vi "BFP-CLAMP-baselinecorrect.vi"() -> ()   [LabVIEW 2017]
uses:
  <vilib>/userdefined/High Color/IMAQdx.ctl
  <vilib>/vision/driver/IMAQdx.llb/IMAQdx Buffer Number Mode.ctl
  <vilib>/DAQmx/write.llb/DAQmx Write (Analog DBL 1Chan 1Samp).vi
  <vilib>/Utility/file.llb/Write To Spreadsheet File (DBL).vi
  <vilib>/Utility/file.llb/Write To Spreadsheet File (string).vi
  <vilib>/DAQmx/create/channels.llb/DAQmx Create Channel (AO-Voltage-Basic).vi
  <vilib>/DAQmx/miscellaneous.llb/DAQmx Fill In Error Info.vi
  <vilib>/Utility/file.llb/Read From Spreadsheet File (DBL).vi
  <vilib>/vision/NI_Vision_Development_Module.lvlib
  <vilib>/vision/driver/NI_Vision_Acquisition_Software.lvlib
  <resource>/objmgr/imaqdx.rc
panel:
  in  "Clamp at (pN)":dbl
  in  "SD x":dbl=1.0
  out "clamp test":bool=TRUE
  out "Data":cluster{"Y":dbl[], "Y":dbl[]}[](graph)
  out "chemin complet force mean":path
  in  "box mean (pts)":i32=10
  out "chemin complet position":path
  out "test fin":bool
  out "t0":u32
  out "slow":string="prosilica-slow.icd"
  out "fast":string="prosilica.icd"
  out "derniere image":u32
  out "chemin complet force":path
  out "chemin":path caption="chemin sélectionné"
  out "# FC":i32
  out "voltage stop (V)":dbl
  out "cluster fit":T1
  out "N pas wait":i32
  out "N pas stop":i32
  in  "F contact (pN)":dbl=500.0
  in  "Measure forces":bool
  in  "Z lenght (um)":dbl=1.0
  in  "v press (um/s)":dbl=1.0
  out "t total / FC (s)":dbl
  out "# pts press":i32=500
  out "DV P753.2DV (V/um)":dbl
  in  "number A/R":i32=5
  out "step press (V)":dbl
  out "step press  (ms)":dbl
  out "V max (V)":dbl
  in  "t contact (s)":dbl
  out "t total / run (s)":dbl
  in  "t wait (s)":dbl=1.0
  in  "v pull (um/s)":dbl=1.0
  out "# pts pull":i32=500
  out "step pull  (ms)":dbl
  out "step pull (V)":dbl
  out "rectangle selection":i32[](array[numeric])
  out "calib um/pix":dbl=0.094 format="%.4f"
  in  "calibration":dbl=0.094
  out "X coord profile":dbl[](array[numeric])
  out "baseline (pN)":dbl caption="B-Line (pN)" format="%0.2f"
  out "SD noise (pN)":dbl caption="SD (pN)" format="%0.2f"
  in  "longueur fit (pts)":i32=11
  out "40x 1.5x 6.7x":dbl=3.0
  out "40x 1x 6.7x":dbl=3.0
  in  "IMAQdx MAZ":T2="cam0"
  out "Frame Rate":dbl
  out "?":T3(plugin-control)
  out "2Rc (µm)":dbl
  out "2Rg (µm)":dbl=8.0
  out "2Rp (µm)":dbl=3.0
  out "DP (cmH2O)":dbl
  in  "2Rc (pix)":dbl=1.0
  in  "2Rg (pix)":dbl=8.0
  in  "2Rp (pix)":dbl=3.0
  in  "k voulue (pN/nm)":dbl=1.0
  in  "Stop calibration":bool
  in  "sortie carte AO":tag="Dev1/ao0" caption="AO"
  in  "IMAQdx Session":T2="cam0"
  out "profil / pix":cluster{dbl[], "X Axis Averages":sgl[]}(graph)
  out "Frame Rate":dbl
  in  "Stop (F) 2":bool caption="Stop focus"
  out "FOCUSING":T3(plugin-control)
  out "ligneY (pix) <=7":i32
  out "ligne X (pix) >=200":i32
  # "Indicateurs variables locales"
  # "CALIBRATION"
  # "CAMERA"
  # "CLAMP"
  # "exposure 1 msec, gain = 24 (set in MAX)"
  # "Noise \nand Baseline\ncorrections"
  # "PIEZO"
  # ">>>"
  # "FORCE PARAMETERS"
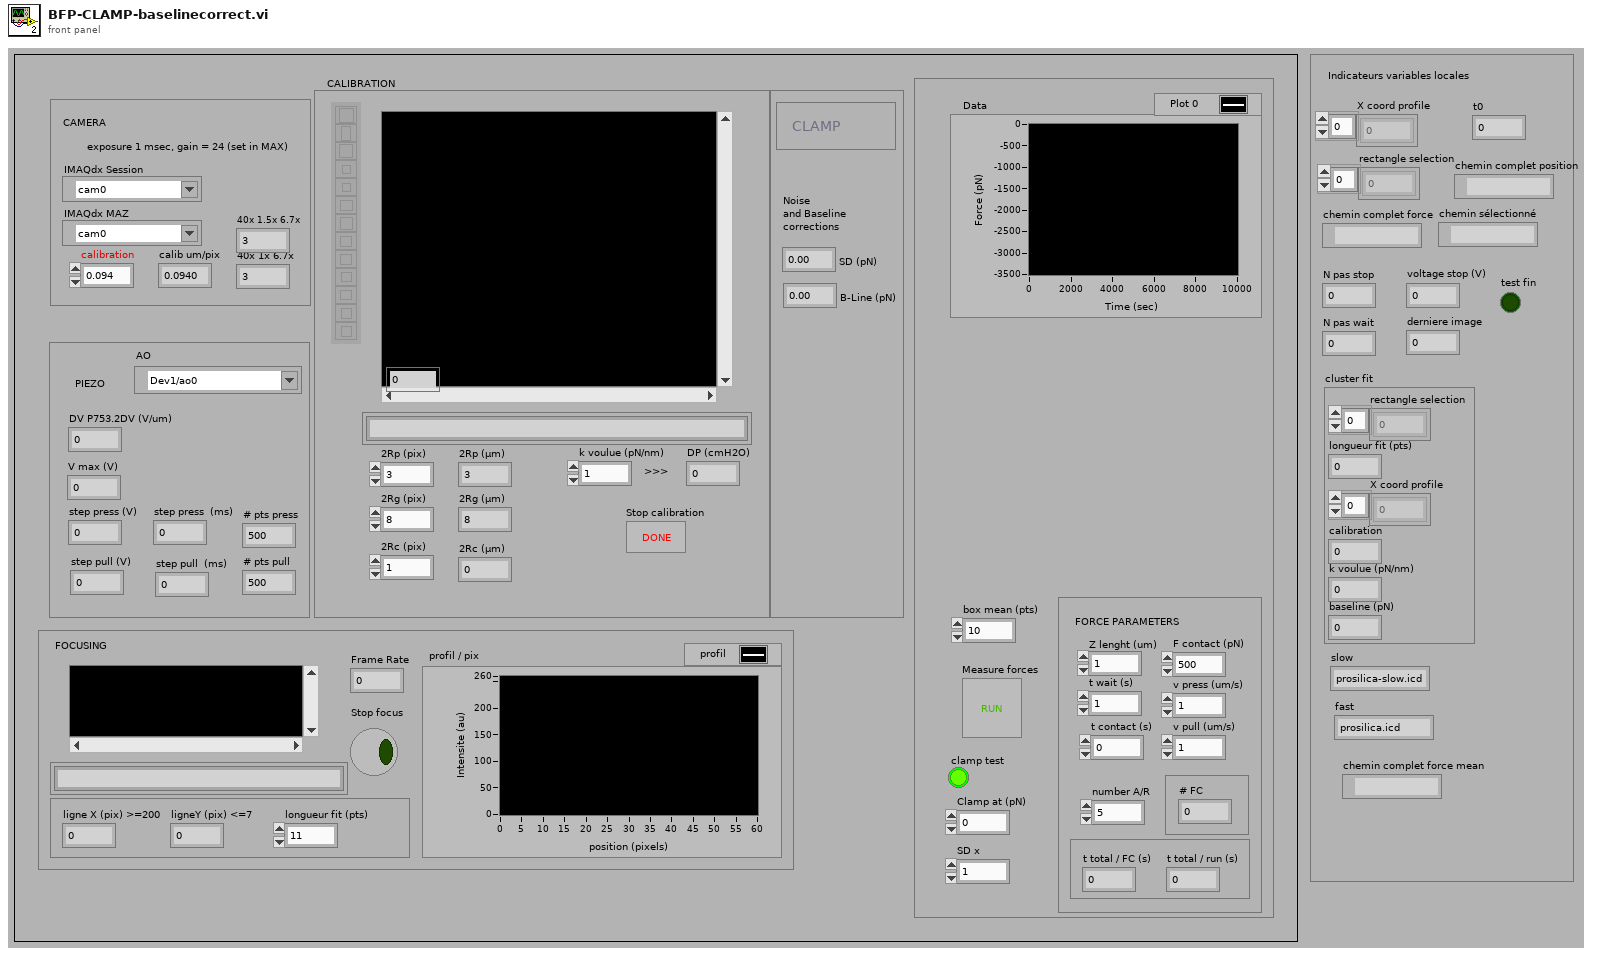
[diagram p1: front panel]
types:
  T1 = cluster{"rectangle selection":i32[], "longueur fit (pts)":i32, "X coord profile":dbl[], "calibration":dbl, "k voulue (pN/nm)":dbl, "baseline (pN)":dbl}
  T2 = typedef "IMAQdx.ctl" = refnum<k21>
  T3 = typedef "IMAQ Image.ctl" = refnum<image>
  T4 = typedef "NI_Vision_Acquisition_Software.lvlib/IMAQdx Buffer Number Mode.ctl" = enum32{"Next", "Last", "Buffer Number", "Every", "Last New"}
  T5 = typedef "IMAQ Rectangle" = cluster{"Left":i32, "Top":i32, "Right":i32, "Bottom":i32, "Rotation":dbl}
  T6 = typedef "ROI Descriptor" = cluster{"Global Rectangle":i32[], "Contours":cluster{"ID":enum32{"External", "Internal"}, "Type":u32, "Coordinates":i32[]}[]}
  T7 = cluster{"Left":i32, "Top":i32, "Right":i32, "Bottom":i32}
  T8 = cluster{"Global Rectangle[0]":i32, "Global Rectangle[1]":i32, "Global Rectangle[2]":i32, "Global Rectangle[3]":i32, "Global Rectangle[4]":i32, "Global Rectangle[5]":i32, "Global Rectangle[6]":i32, "Global Rectangle[7]":i32, "Global Rectangle[8]":i32}
  T9 = cluster{"task out":refnum<k21>, "error out":errorcluster}
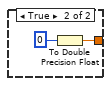
[diagram p4: hidden frame]
diagram:
  n1 = flat-sequence {
    tunnel: [w72] -> w13
    tunnel: w13 -> [w84]
    tunnel: [w161] -> w6
    tunnel: [w160] -> w4
    tunnel: [w159] -> w2
    tunnel: w6 -> [w245]
    tunnel: [w245] -> w5
    tunnel: w4 -> [w244]
    tunnel: [w244] -> w3
    tunnel: w2 -> [w243]
    tunnel: [w243] -> w1
    tunnel: w5 -> [w258]
    tunnel: w3 -> [w248]
    tunnel: w1 -> [w249]
    tunnel: [w246] -> w12
    tunnel: [w247] -> w10
    tunnel: [w250] -> w8
    tunnel: w12 -> [w270]
    tunnel: [w270] -> w11
    tunnel: w10 -> [w269]
    tunnel: [w269] -> w9
    tunnel: w8 -> [w268]
    tunnel: [w268] -> w7
    tunnel: w11 -> [w277]
    tunnel: w9 -> [w274]
    tunnel: w7 -> [w275]
    frame #0 {
      n2 = call <vilib>:"IMAQdx Open Camera.vi"("Session In"="IMAQdx MAZ") -> ("error out"=w21:errorcluster, "Session Out"=w20:T2)  [unwired: 2 in, 7 out]
      n3 = call <vilib>:"IMAQdx Read Attributes.vi"("error in"=w21, "Filename"="defaut.icd", "Session In"=w20) -> ("error out"=w19:errorcluster, "Session Out"=w24:T2)  [unwired: 7 out]
      n4 = call <vilib>:"IMAQdx Configure Grab.vi"("error in"=w19, "Session In"=w24) -> ("error out"=w16:errorcluster, "Session Out"=w17:T2)  [unwired: 1 in, 7 out]
      n5 = call <vilib>:"IMAQdx Close Camera.vi"("error in"=w16, "Session In"=w17) -> ("error out"=w18:errorcluster)  [unwired: 9 out]
      n6 = call <vilib>:"Simple Error Handler.vi"("error in (no error)"=w18) -> ()  [unwired: 1 in, 8 out]
      "40x 1x 6.7x" <- ext 0.094 ("40x 1x 6.7x")
      "40x 1.5x 6.7x" <- ext 0.0625 ("40x 1x 6.7x")
    }
    frame #1 {
      n7 = while "calibration \"evans\"" {
        stop <- w29 stop-if-true
        n8 = local write "calibration"("calibration") -> ()
        n9 = Bundle(240, 251, 440, 230) -> (w33:cluster{i32, i32, i32, i32})  [unwired: 1 out]
        n10 = Multiply(x="calibration", y="2Rc (pix)") -> (x*y=w40:dbl)
        "2Rc (µm)" <- w40
        n11 = Multiply(x="2Rp (pix)", y="calibration") -> (x*y=w44:dbl)
        "2Rp (µm)" <- w44
        n12 = Multiply(x="2Rg (pix)", y="calibration") -> (x*y=w41:dbl)
        "2Rg (µm)" <- w41
        n13 = Divide(x=1, y=1000000) -> (x/y=w66:dbl)
        n14 = Divide(x=3.141592653589793, y=2) -> (x/y=w52:dbl)
        n15 = Divide(x=1, y=1000) -> (x/y=w67:dbl)
        n16 = local write "k voulue (pN/nm)"("k voulue (pN/nm)") -> ()
        n17 = call "Vision Acquisition"("Stop (F)"="Stop calibration") -> ("Image Out"=w31:T3, "Frame Rate"=→"Frame Rate":dbl, "Stopped"=w29:bool)  [unwired: 3 in, 21 out]
        n18 = Multiply(x="k voulue (pN/nm)", y=w67) -> (x*y=w64:dbl)
        n19 = Multiply(x=w52, y=w66) -> (x*y=w65:dbl)
        n20 = Divide(x=w41, y=w40) -> (x/y=w39:dbl)
        n21 = Divide(x=w41, y=w44) -> (x/y=w43:dbl)
        n22 = Multiply(x=w44, y=w65) -> (x*y=w47:dbl)
        n23 = call "IMAQ Overlay Rectangle"("Rectangle"=w33, "Image"=w31) -> ("Image Out"=→"?":T3)  [unwired: 4 in, 5 out]
        n24 = Multiply(x=w39, y=2) -> (x*y=w59:dbl)
        n25 = Multiply(x=2, y=w43) -> (x*y=w62:dbl)
        n26 = Reciprocal(x=w43) -> (1/x=w42:dbl)
        n27 = Natural Logarithm(1:w59) -> (0:w57:dbl)
        n28 = Natural Logarithm(1:w62) -> (0:w58:dbl)
        n29 = Add(x=w57, y=w58) -> (x+y=w55:dbl)
        n30 = Subtract(x=1, y=w42) -> (x-y=w56:dbl)
        n31 = Multiply(x=w56, y=w55) -> (x*y=w38:dbl)
        n32 = Divide(x=w47, y=w38) -> (x/y=w46:dbl)
        n33 = Divide(x=w64, y=w46) -> (x/y=w50:dbl)
        n34 = Multiply(x=w50, y=0.010197) -> (x*y=w26:dbl)
        "DP (cmH2O)" <- w26
        n35 = local write "DP (cmH2O)"(w26) -> ()
        "calib um/pix" <- "calibration"
      }
    }
    frame #2 {
      n36 = while "focusing 100 fps" {
        tunnel: [w73] -> w72
        stop <- w75 stop-if-true
        n37 = call "Vision Acquisition3"("Stop (F)"="Stop (F) 2") -> ("Image Out"=w73:T3, "Frame Rate"=→"Frame Rate":dbl, "Stopped"=w75:bool)  [unwired: 1 in, 23 out]
        "FOCUSING" <- w73
      }
    }
    frame #3 {
      w86 = i32[] [0, 1] items=["X Axis Averages", "Y Axis Averages", "X + Y Axis Averages", "X - Y Axis Averages"] ("Averages")
      n38 = call "IMAQ Select Rectangle"("Image In"=w84) -> ("Rectangle"=w99:T5)  [unwired: 4 in, 6 out]
      n39 = Unbundle(w99) -> ("Left"=w91:i32, "Top"=w90:i32, "Right"=w89:i32, "Bottom"=w88:i32)  [unwired: 1 out]
      n40 = call "IMAQ Convert Rectangle to ROI"("Rectangle"=w99) -> ("ROI Descriptor"=w80:T6)  [unwired: 1 in, 8 out]
      n41 = Bundle("Left"=w91, "Top"=w90, "Right"=w89, "Bottom"=w88) -> (w87:T7)  [unwired: 1 out]
      n42 = Unbundle(w80) -> ("Global Rectangle"=w104:i32[])  [unwired: 1 out]
      n43 = Cluster To Array(cluster=w87) -> (array=w82:i32[])
      "rectangle selection" <- w82
      n44 = Array To Cluster(array=w104) -> (cluster=w103:T8)
      n45 = local write "rectangle selection"(w82) -> ()
      n46 = call "IMAQ LinearAverages"("Averages"=w86, "Optional Rectangle"=w82, "Image Src"=w84) -> ("X Axis Averages"=w85:sgl[])  [unwired: 1 in, 7 out]
      n47 = Unbundle(w103) -> ("Global Rectangle[0]"=w102:i32, "Global Rectangle[1]"=w97:i32, "Global Rectangle[2]"=w101:i32, "Global Rectangle[3]"=w96:i32)  [unwired: 5 out]
      n48 = Subtract(x=w102, y=w101) -> (x-y=w100:i32)
      n49 = Subtract(x=w97, y=w96) -> (x-y=w98:i32)
      n50 = Absolute Value(x=w100) -> (abs(x)=w78:i32)
      "ligne X (pix) >=200" <- w78
      n51 = Absolute Value(x=w98) -> (abs(x)=w79:i32)
      "ligneY (pix) <=7" <- w79
      n52 = local write "ligne X (pix) >=200"(w78) -> ()
      n53 = local write "ligneY (pix) <=7"(w79) -> ()
      n54 = Subtract(x=w78, y=1) -> (x-y=w81:i32)
      n55 = Initialize Array(0.0 ("élément"), 1 ("taille de la dimension")) -> (w92:dbl[])
      n56 = for {
        N: w81 -> [_]
        shift-right: [w109] -> w83
        shift-left: w92 -> [w108]
        i -> [w107]
        n57 = Add(x=1, y=w107) -> (x+y=w106:i32)
        n58 = Build Array (concatenate)(w108, w106) -> (w109:dbl[])
      }
      "X coord profile" <- w83
      n59 = local write "X coord profile"(w83) -> ()
      n60 = Bundle(w83, "X Axis Averages"=w85) -> (w77:cluster{dbl[], "X Axis Averages":sgl[]})  [unwired: 1 out]
      "profil / pix" <- w77
      n61 = local write "profil / pix"(w77) -> ()
    }
    frame #4 {
      n62 = while {
        stop <- "Measure forces" stop-if-true
        w124 = 2
        w123 = 2
        w125 = 0.4  # DV P753.2DV (V/um)
        n63 = local write "F contact (pN)"("F contact (pN)") -> ()
        n64 = local write "v pull (um/s)"("v pull (um/s)") -> ()
        n65 = local write "step pull  (ms)"(w123) -> ()
        n66 = local write "number A/R"("number A/R") -> ()
        n67 = local write "step press  (ms)"(w124) -> ()
        n68 = local write "t contact (s)"("t contact (s)") -> ()
        n69 = local write "t wait (s)"("t wait (s)") -> ()
        n70 = local write "SD x"("SD x") -> ()
        n71 = Divide(x="Z lenght (um)", y="v pull (um/s)") -> (x/y=w114:dbl)
        n72 = Divide(x="Z lenght (um)", y="v press (um/s)") -> (x/y=w113:dbl)
        n73 = Multiply(x="t wait (s)", y=1000.0) -> (x*y=w130:dbl)
        n74 = Multiply(x=1000, y="t contact (s)") -> (x*y=w137:dbl)
        n75 = local write "Clamp at (pN)"("Clamp at (pN)") -> ()
        n76 = local write "box mean (pts)"("box mean (pts)") -> ()
        n77 = Divide(x=w130, y=w123) -> (x/y=w129:dbl)
        n78 = Add(x="t contact (s)", y=w114) -> (x+y=w143:dbl)
        n79 = Divide(x=w137, y=w124) -> (x/y=w146:dbl)
        n80 = Multiply(x=1000, y=w114) -> (x*y=w118:dbl)
        n81 = Multiply(x=1000, y=w113) -> (x*y=w121:dbl)
        n82 = local write "DV P753.2DV (V/um)"(w125) -> ()
        n83 = Add(x=w143, y=w113) -> (x+y=w127:dbl)
        n84 = Multiply(x="Z lenght (um)", y=w125) -> (x*y=w138:dbl)
        "V max (V)" <- w138
        n85 = To Long Integer(number=w129) -> (32bit integer=w128:i32)
        "N pas wait" <- w128
        n86 = To Long Integer(number=w146) -> (32bit integer=w133:i32)
        "N pas stop" <- w133
        n87 = Divide(x=w118, y=2) -> (x/y=w115:dbl)
        "# pts pull" <- w115
        n88 = Divide(x=w121, y=2) -> (x/y=w119:dbl)
        "# pts press" <- w119
        n89 = local write "N pas stop"(w133) -> ()
        n90 = local write "# pts pull"(w115) -> ()
        n91 = local write "N pas wait"(w128) -> ()
        n92 = local write "V max (V)"(w138) -> ()
        n93 = local write "# pts press"(w119) -> ()
        n94 = Divide(x="Z lenght (um)", y=w115) -> (x/y=w141:dbl)
        n95 = Divide(x="Z lenght (um)", y=w119) -> (x/y=w148:dbl)
        n96 = Add(x=w127, y="t wait (s)") -> (x+y=w144:dbl)
        "t total / FC (s)" <- w144
        n97 = Multiply(x=w144, y="number A/R") -> (x*y=→"t total / run (s)":dbl)
        n98 = Multiply(x=w141, y=w125) -> (x*y=w139:dbl)
        "step pull (V)" <- w139
        n99 = Multiply(x=w148, y=w125) -> (x*y=w140:dbl)
        "step press (V)" <- w140
        n100 = local write "step pull (V)"(w139) -> ()
        n101 = local write "step press (V)"(w140) -> ()
        "DV P753.2DV (V/um)" <- w125
        "step press  (ms)" <- w124
        "step pull  (ms)" <- w123
      }
    }
    frame #5 {
      w153 = "force"  # default name
      w151 = "prosilica.icd" ("Filename")
      n102 = local write "fast"(w151) -> ()
      n103 = call "Boîte de dialogue de fichier"("default name"=w153) -> ("selected path"=w152:path)  [unwired: 6 in, 8 out]
      "chemin" <- w152
      n104 = call "IMAQ Create"("Image Name"="IMAQdx Session") -> ("New Image"=w159:T3)  [unwired: 3 in, 2 out]
      n105 = call <vilib>:"IMAQdx Open Camera.vi"("Session In"="IMAQdx Session") -> ("error out"=w156:errorcluster, "Session Out"=w157:T2)  [unwired: 2 in, 7 out]
      n106 = local write "chemin"(w152) -> ()
      n107 = call <vilib>:"IMAQdx Read Attributes.vi"("error in"=w156, "Filename"=w151, "Session In"=w157) -> ("error out"=w155:errorcluster, "Session Out"=w154:T2)  [unwired: 7 out]
      n108 = call <vilib>:"IMAQdx Configure Grab.vi"("error in"=w155, "Session In"=w154) -> ("error out"=w161:errorcluster, "Session Out"=w160:T2)  [unwired: 1 in, 7 out]
      "fast" <- w151
    }
    frame #6 {
      w168 = FALSE
      n109 = local read "v press (um/s)"() -> (w177:dbl)
      n110 = local read "Z lenght (um)"() -> (w173:dbl)
      n111 = local read "v pull (um/s)"() -> (w172:dbl)
      n112 = local read "profil / pix"() -> (w187:cluster{dbl[], "X Axis Averages":sgl[]})
      n113 = local read "chemin"() -> (w191:path)
      n114 = Get Date/Time String() -> (date string=w202:string, time string=w200:string)  [unwired: 3 out]
      n115 = local write "clamp test"(w168) -> ()
      n116 = Concatenate Strings(w202, "   ", w200) -> (w201:string)
      n117 = Divide(x=w173, y=w177) -> (x/y=w178:dbl)
      n118 = Divide(x=w173, y=w172) -> (x/y=w174:dbl)
      n119 = Unbundle(w187) -> (w186:dbl[], "X Axis Averages"=w185:sgl[])
      n120 = Strip Path(path=w191) -> (stripped path=w184:path, name=w183:string)
      n121 = Build Array(w186, w185) -> (w182:dbl[][])
      n122 = Concatenate Strings("data-clamp-", w183, ".txt" ("chaîne")) -> (w214:string)
      n123 = Concatenate Strings("profile-", w183, ".txt" ("chaîne")) -> (w194:string)
      n124 = Multiply(x=1000, y=w178) -> (x*y=w180:dbl)
      n125 = Multiply(x=1000, y=w174) -> (x*y=w170:dbl)
      n126 = Insert Into Array(array=string[] [] ("tableau"), new element #1=w201, new element #2="calibration (um/pix)", new element #3="k (pN/nm)", new element #4="2Rc (um)", new element #5="2Rp (um)", new element #6="2Rg(um)", new element #7="fit x (pix)", new element #8="fit y (pix)", new element #9="# FC", new element #10="t wait (s)", new element #11="v A (um/s)", new element #12="# pts A", new element #13="t contact (s)", new element #14="F contact (pN)", new element #15="v R (um/s)", new element #16="# pts R", new element #17="Z lentgh (um)", new element #18="DP (cmH20)" ("nouvel élément/sous-tableau"), new element #19="F clamp (pN)" ("nouvel élément/sous-tableau"), new element #20="SD x" ("nouvel élément/sous-tableau"), new element #21="F contact (pN)" ("nouvel élément/sous-tableau")) -> (w210:string[])  [unwired: 1 in]
      n127 = local read "ligne X (pix) >=200"() -> (w226:i32)
      n128 = local read "k voulue (pN/nm)"() -> (w217:dbl)
      n129 = local read "F contact (pN)"() -> (w162:dbl)
      n130 = local read "ligneY (pix) <=7"() -> (w225:i32)
      n131 = local read "F contact (pN)"() -> (w221:dbl)
      n132 = Build Path(base path=w184, name or relative path=w214) -> (appended path=w211:path)
      n133 = Build Path(base path=w184, name or relative path=w194) -> (appended path=w188:path)
      n134 = local read "DP (cmH2O)"() -> (w205:dbl)
      n135 = local read "number A/R"() -> (w224:i32)
      n136 = local read "t contact (s)"() -> (w222:dbl)
      n137 = local read "calibration"() -> (w216:dbl)
      n138 = local read "2Rp (µm)"() -> (w219:dbl)
      n139 = local read "2Rg (µm)"() -> (w220:dbl)
      n140 = local read "2Rc (µm)"() -> (w218:dbl)
      n141 = local read "Clamp at (pN)"() -> (w165:dbl)
      n142 = local read "t wait (s)"() -> (w223:dbl)
      n143 = Quotient & Remainder(x=w180, y=2) -> (floor(x/y)=w176:dbl)  [unwired: 1 out]
      n144 = Quotient & Remainder(x=w170, y=2) -> (floor(x/y)=w169:dbl)  [unwired: 1 out]
      n145 = local read "SD x"() -> (w164:dbl)
      n146 = local write "# pts pull"(w169) -> ()
      n147 = local write "# pts press"(w176) -> ()
      n148 = call-poly <vilib>:"Write To Spreadsheet File.vi"("transpose? (no:F)"=TRUE, "append to file? (new file:F)"=FALSE, "2D data"=w182, "file path (dialog if empty)"=w188) -> ()  [unwired: 2 in, 3 out]
      n149 = Insert Into Array(array=dbl[] [] ("tableau"), new element #1=0.0 ("nouvel élément/sous-tableau"), new element #2=w216, new element #3=w217, new element #4=w218, new element #5=w219, new element #6=w220, new element #7=w226, new element #8=w225, new element #9=w224, new element #10=w223, new element #11=w177, new element #12=w176, new element #13=w222, new element #14=w221, new element #15=w172, new element #16=w169, new element #17=w173, new element #18=w205, new element #19=w165, new element #20=w164, new element #21=w162) -> (w209:dbl[])  [unwired: 1 in]
      n150 = Number To Fractional String(number=w209, width (-)=i16 10 ("largeur (-)"), precision (6)=i16 3 ("largeur (-)")) -> (F-format string=w207:string[])  [unwired: 1 out]
      n151 = Build Array(w210, w207) -> (w208:string[][])
      n152 = call-poly <vilib>:"Write To Spreadsheet File.vi"("transpose? (no:F)"=TRUE, "append to file? (new file:F)"=FALSE, "2D data"=w208, "file path (dialog if empty)"=w211) -> ()  [unwired: 2 in, 3 out]
      "clamp test" <- w168
    }
    frame #7 {
      n153 = local read "X coord profile"() -> (w256:dbl[])
      n154 = local read "calibration"() -> (w255:dbl)
      n155 = local read "rectangle selection"() -> (w257:i32[])
      n156 = local read "k voulue (pN/nm)"() -> (w254:dbl)
      n157 = local read "longueur fit (pts)"() -> (w253:i32)
      n158 = local write "longueur fit (pts)"("longueur fit (pts)") -> ()
      n159 = call "baseline.vi"("N"=1000, "X coord profile"=w256, "calibration"=w255, "New Image"=w249, "Session Out"=w248, "error out"=w258, "rectangle selection"=w257, "k voulue (pN/nm)"=w254, "longueur fit (pts)"=w253) -> ("baseline"=w252:dbl, "sd"=w251:dbl, "Image Out"=w247:T3, "Session Out 2"=w246:T2, "error out 2"=w250:errorcluster)  [unwired: 2 out]
      "SD noise (pN)" <- w251
      "baseline (pN)" <- w252
      n160 = local write "baseline (pN)"(w252) -> ()
      n161 = local write "SD noise (pN)"(w251) -> ()
    }
    frame #8 {
      n162 = local read "X coord profile"() -> (w265:dbl[])
      n163 = local read "baseline (pN)"() -> (w262:dbl)
      n164 = local read "rectangle selection"() -> (w267:i32[])
      n165 = local read "k voulue (pN/nm)"() -> (w263:dbl)
      n166 = local read "longueur fit (pts)"() -> (w266:i32)
      n167 = local read "calibration"() -> (w264:dbl)
      n168 = Bundle("rectangle selection"=w267, "longueur fit (pts)"=w266, "X coord profile"=w265, "calibration"=w264, "k voulue (pN/nm)"=w263, "baseline (pN)"=w262) -> (w261:T1)  [unwired: 1 out]
      "cluster fit" <- w261
      n169 = local write "cluster fit"(w261) -> ()
    }
    frame #9 {
      n170 = call-poly <vilib>:"DAQmx Create Virtual Channel.vi"("maximum value"=10.0, "minimum value"=-10.0, "physical channels"="sortie carte AO") -> ("task out"=w282:refnum<k21>, "error out"=w281:errorcluster)  [unwired: 6 in, 5 out]
      n171 = call <vilib>:"DAQmx Start Task.vi"("task/channels in"=w282, "error in"=w281) -> ("task out"=w279:refnum<k21>, "error out"=w280:errorcluster)  [unwired: 12 out]
      n172 = flat-sequence {
        tunnel: w279 -> [w294]
        tunnel: w280 -> [w292]
        tunnel: [w291] -> w287
        tunnel: [w293] -> w286
        tunnel: [w290] -> w278
        tunnel: w277 -> [w290]
        tunnel: [w289] -> w276
        tunnel: w275 -> [w289]
        tunnel: w287 -> [w304]
        tunnel: w286 -> [w303]
        tunnel: w278 -> [w301]
        tunnel: w276 -> [w300]
        tunnel: w274 -> [w299]
        tunnel: [w298] -> w273
        tunnel: [w297] -> w272
        tunnel: [w296] -> w271
        tunnel: w273 -> [w832]
        tunnel: w272 -> [w829]
        tunnel: w271 -> [w828]
        frame #0 {
          w288 = "prosilica-slow.icd" ("Filename")
          n173 = local write "slow"(w288) -> ()
          n174 = call-poly <vilib>:"DAQmx Write.vi"("task/channels in"=w294, "data"=0.0, "error in"=w292) -> ("task out"=w293:refnum<k21>, "error out"=w291:errorcluster)  [unwired: 1 in, 10 out]
          "slow" <- w288
        }
        frame #1 {
          n175 = local read "number A/R"() -> (w302:i32)
          n176 = for {
            N: w302 -> [_]
            tunnel: w304 -> [w349]
            tunnel: w303 -> [w348]
            tunnel: w301 -> [w347]
            tunnel: w300 -> [w346]
            tunnel: w299 -> [w345]
            tunnel: [w338] -> w298
            tunnel: [w328] -> w297
            tunnel: [w326] -> w296
            i -> [w335]
            n177 = flat-sequence "piezo : stop / run / stop / run" {
              tunnel: w349 -> [w364]
              tunnel: w348 -> [w365]
              tunnel: w347 -> [w353]
              tunnel: w346 -> [w351]
              tunnel: w345 -> [w355]
              tunnel: w335 -> [w366]
              tunnel: [w366] -> w310
              tunnel: [w354] -> w309
              tunnel: [w350] -> w308
              tunnel: [w352] -> w307
              tunnel: [w365] -> w306
              tunnel: [w364] -> w305
              tunnel: [w379] -> w316
              tunnel: [w378] -> w315
              tunnel: [w377] -> w314
              tunnel: [w376] -> w313
              tunnel: [w375] -> w312
              tunnel: [w374] -> w311
              tunnel: w310 -> [w379]
              tunnel: w309 -> [w378]
              tunnel: w308 -> [w377]
              tunnel: w307 -> [w376]
              tunnel: w306 -> [w375]
              tunnel: w305 -> [w374]
              tunnel: [w409] -> w333
              tunnel: [w408] -> w332
              tunnel: [w407] -> w331
              tunnel: [w406] -> w330
              tunnel: [w405] -> w329
              tunnel: w316 -> [w396]
              tunnel: w315 -> [w405]
              tunnel: w314 -> [w406]
              tunnel: w313 -> [w407]
              tunnel: w312 -> [w408]
              tunnel: w311 -> [w409]
              tunnel: [w420] -> w344
              tunnel: [w419] -> w343
              tunnel: [w418] -> w340
              tunnel: [w414] -> w337
              tunnel: w333 -> [w416]
              tunnel: w332 -> [w417]
              tunnel: w331 -> [w410]
              tunnel: w330 -> [w413]
              tunnel: w329 -> [w425]
              tunnel: w344 -> [w539]
              tunnel: w343 -> [w538]
              tunnel: [w537] -> w342
              tunnel: [w536] -> w341
              tunnel: w340 -> [w535]
              tunnel: [w534] -> w339
              tunnel: w337 -> [w533]
              tunnel: [w532] -> w336
              tunnel: w342 -> [w605]
              tunnel: w341 -> [w602]
              tunnel: [w604] -> w324
              tunnel: [w603] -> w322
              tunnel: w339 -> [w601]
              tunnel: [w600] -> w320
              tunnel: w336 -> [w599]
              tunnel: [w598] -> w318
              tunnel: w324 -> [w700]
              tunnel: [w700] -> w323
              tunnel: w322 -> [w699]
              tunnel: [w699] -> w321
              tunnel: w320 -> [w698]
              tunnel: [w698] -> w319
              tunnel: w318 -> [w697]
              tunnel: [w697] -> w317
              tunnel: w323 -> [w710]
              tunnel: w321 -> [w704]
              tunnel: w319 -> [w718]
              tunnel: w317 -> [w709]
              tunnel: [w717] -> w334
              tunnel: [w703] -> w327
              tunnel: [w702] -> w325
              tunnel: w334 -> [w827]
              tunnel: [w827] -> w338
              tunnel: [w817] -> w328
              tunnel: w327 -> [w817]
              tunnel: [w816] -> w326
              tunnel: w325 -> [w816]
              frame #0 {
                n178 = local read "rectangle selection"() -> (w362:i32[])
                n179 = local read "k voulue (pN/nm)"() -> (w359:dbl)
                n180 = local read "longueur fit (pts)"() -> (w358:i32)
                n181 = local read "X coord profile"() -> (w361:dbl[])
                n182 = local read "calibration"() -> (w360:dbl)
                n183 = call "baseline.vi"("N"=1000, "X coord profile"=w361, "calibration"=w360, "New Image"=w355, "Session Out"=w353, "error out"=w351, "rectangle selection"=w362, "k voulue (pN/nm)"=w359, "longueur fit (pts)"=w358) -> ("baseline"=w357:dbl, "sd"=w356:dbl, "Image Out"=w354:T3, "Session Out 2"=w352:T2, "error out 2"=w350:errorcluster)  [unwired: 2 out]
                n184 = local write "baseline (pN)"(w357) -> ()
                n185 = local write "SD noise (pN)"(w356) -> ()
              }
              frame #1 {
                n186 = local read "X coord profile"() -> (w371:dbl[])
                n187 = local read "baseline (pN)"() -> (w368:dbl)
                n188 = local read "rectangle selection"() -> (w373:i32[])
                n189 = local read "k voulue (pN/nm)"() -> (w369:dbl)
                n190 = local read "longueur fit (pts)"() -> (w372:i32)
                n191 = local read "calibration"() -> (w370:dbl)
                n192 = Bundle("rectangle selection"=w373, "longueur fit (pts)"=w372, "X coord profile"=w371, "calibration"=w370, "k voulue (pN/nm)"=w369, "baseline (pN)"=w368) -> (w367:T1)  [unwired: 1 out]
                n193 = local write "cluster fit"(w367) -> ()
              }
              frame #2 {
                w386 = ".txt"
                n194 = local read "chemin"() -> (w400:path)
                n195 = local read "chemin"() -> (w393:path)
                n196 = Add(x=1, y=w396) -> (x+y=w403:i32)
                "# FC" <- w403
                n197 = Add(x=1, y=w396) -> (x+y=w394:i32)
                n198 = Strip Path(path=w393) -> (stripped path=w398:path, name=w390:string)
                n199 = Number To Decimal String(number=w394) -> (decimal integer string=w388:string)  [unwired: 1 out]
                n200 = Strip Path(path=w400) -> (stripped path=w382:path, name=w385:string)
                n201 = Number To Decimal String(number=w403) -> (decimal integer string=w384:string)  [unwired: 1 out]
                n202 = Concatenate Strings(w385, "-mean-", w384, w386) -> (w381:string)
                n203 = Concatenate Strings(w385, "-", w384, w386) -> (w401:string)
                n204 = Concatenate Strings("voltage-", w390, "-", w388, ".txt") -> (w397:string)
                n205 = Build Path(base path=w382, name or relative path=w381) -> (appended path=w380:path)
                "chemin complet force mean" <- w380
                n206 = Build Path(base path=w382, name or relative path=w401) -> (appended path=w399:path)
                "chemin complet force" <- w399
                n207 = local write "chemin complet force mean"(w380) -> ()
                n208 = local write "chemin complet force"(w399) -> ()
                n209 = Build Path(base path=w398, name or relative path=w397) -> (appended path=w392:path)
                "chemin complet position" <- w392
                n210 = local write "chemin complet position"(w392) -> ()
              }
              frame #3 {
                w431 = 2
                n211 = local read "t wait (s)"() -> (w427:dbl)
                n212 = Bundle("task out"=w417, "error out"=w416) -> (w415:T9)  [unwired: 1 out]
                n213 = local read "fast"() -> (w412:string)
                n214 = Tick Count (ms)() -> (millisecond timer value=w411:u32)
                "t0" <- w411
                n215 = local write "t0"(w411) -> ()
                n216 = call <vilib>:"IMAQdx Read Attributes.vi"("error in"=w413, "Filename"=w412, "Session In"=w410) -> ("error out"=w423:errorcluster, "Session Out"=w424:T2)  [unwired: 7 out]
                n217 = Multiply(x=w427, y=1000) -> (x*y=w432:dbl)
                n218 = Divide(x=w432, y=w431) -> (x/y=w428:dbl)
                n219 = call <vilib>:"IMAQdx Configure Grab.vi"("error in"=w423, "Session In"=w424) -> ("error out"=w421:errorcluster, "Session Out"=w422:T2)  [unwired: 1 in, 7 out]
                n220 = To Long Integer(number=w428) -> (32bit integer=w426:i32)
                n221 = Not Equal?(x=w428, y=0.0) -> (x != y?=w430:bool)
                n222 = case "si t=o ou non" shown="True" w430 {
                  tunnel: w426 -> [_ w451]
                  tunnel: w431 -> [_ w449]
                  tunnel: w425 -> [w434 w453]
                  tunnel: w422 -> [w437 w460]
                  tunnel: w421 -> [w436 w459]
                  tunnel: [w437 w458] -> w420
                  tunnel: [w436 w457] -> w419
                  tunnel: [w435 w456] -> w418
                  tunnel: w415 -> [w435 w455]
                  tunnel: [w434 w452] -> w414
                  frame False {
                  }
                  frame True {
                    n223 = local read "cluster fit"() -> (w461:T1)
                    n224 = local read "chemin complet position"() -> (w438:path)
                    n225 = while {
                      tunnel: w461 -> [w488]
                      tunnel: w460 -> [w486]
                      tunnel: w459 -> [w484]
                      tunnel: [w483] -> w458
                      tunnel: [w482] -> w457
                      tunnel: [w481] -> w456
                      tunnel: w455 -> [w479]
                      tunnel: 0 -> [w478]
                      tunnel: 0 -> [w477]
                      tunnel: w453 -> [w475]
                      tunnel: [w473] -> w452
                      tunnel: w451 -> [w470]
                      tunnel: w449 -> [w468]
                      tunnel: [w465] -> w448 mode=indexing
                      tunnel: [w464] -> w440 mode=indexing
                      tunnel: [w463] -> w441 mode=indexing
                      i -> [w466]
                      stop <- w469 continue-if-true
                      n226 = Wait Until Next ms Multiple(millisecond multiple=w468) -> ()  [unwired: 1 out]
                      n227 = Bundle(w466, w478, w477) -> (w476:cluster{i32, i32, i32})  [unwired: 1 out]
                      n228 = flat-sequence {
                        tunnel: [w498] -> w487
                        tunnel: w486 -> [w498]
                        tunnel: [w497] -> w485
                        tunnel: w484 -> [w497]
                        tunnel: [w496] -> w480
                        tunnel: w479 -> [w495]
                        tunnel: w476 -> [w494]
                        tunnel: w475 -> [w493]
                        tunnel: [w493] -> w474
                        tunnel: [w492] -> w472
                        tunnel: w466 -> [w492]
                        tunnel: [w491] -> w471
                        tunnel: w470 -> [w491]
                        tunnel: [w490] -> w467
                        tunnel: w466 -> [w490]
                        tunnel: [w489] -> w462
                        tunnel: w488 -> [w517]
                        tunnel: w487 -> [w516]
                        tunnel: w485 -> [w515]
                        tunnel: [w513] -> w483
                        tunnel: [w511] -> w482
                        tunnel: [w510] -> w481
                        tunnel: w480 -> [w510]
                        tunnel: w474 -> [w509]
                        tunnel: [w508] -> w473
                        tunnel: w472 -> [w506]
                        tunnel: w471 -> [w505]
                        tunnel: [w501] -> w469
                        tunnel: w467 -> [_]
                        tunnel: [w504] -> w465
                        tunnel: [w503] -> w464
                        tunnel: [w499] -> w463
                        tunnel: w462 -> [w499]
                        frame #0 {
                          n229 = call "piezo-cluster.vi"("cluster carte entree"=w495, "cluster carte data"=w494) -> ("cluster carte sortie"=w496:T9, "voltage (V)"=w489:dbl)
                        }
                        frame #1 {
                          n230 = Less?(x=w506, y=w505) -> (x < y?=w501:bool)
                          n231 = Tick Count (ms)() -> (millisecond timer value=w502:u32)
                          n232 = local read "t0"() -> (w500:u32)
                          n233 = call <vilib>:"IMAQdx Get Image.vi"("Buffer Number Mode (Next)"=IMAQdx_Buffer_Number_Mode."Next", "error in"=w515, "Image In"=w509, "Session In"=w516) -> ("error out"=w512:errorcluster, "Image Out"=w508:T3, "Session Out"=w514:T2)  [unwired: 1 in, 4 out]
                          n234 = Subtract(x=w502, y=w500) -> (x-y=w503:u32)
                          n235 = property class="IMAQdx" props=["LastBufferNumber"](reference=w514, error in=w512) -> (reference out=w513:T2, error out=w511:errorcluster)  [unwired: 1 out]
                          n236 = call "fit-cluster.vi"("Image In"=w508, "donnees fit"=w517) -> ("F - baseline  (pN)"=w504:dbl)
                        }
                      }
                    }
                    n237 = local read "chemin complet force"() -> (w445:path)
                    n238 = Build Array(w440, w441) -> (w439:dbl[][])
                    n239 = Build Array(w440, w448) -> (w447:dbl[][])
                    n240 = call-poly <vilib>:"Write To Spreadsheet File.vi"("transpose? (no:F)"=TRUE, "append to file? (new file:F)"=FALSE, "2D data"=w439, "file path (dialog if empty)"=w438) -> ()  [unwired: 2 in, 3 out]
                    n241 = call-poly <vilib>:"Write To Spreadsheet File.vi"("transpose? (no:F)"=TRUE, "append to file? (new file:F)"=FALSE, "2D data"=w447, "file path (dialog if empty)"=w445) -> ()  [unwired: 2 in, 3 out]
                  }
                }
              }
              frame #4 {
                n242 = local read "step press  (ms)"() -> (w529:dbl)
                n243 = local read "step press (V)"() -> (w531:dbl)
                n244 = local read "cluster fit"() -> (w540:T1)
                n245 = while {
                  tunnel: w540 -> [w565]
                  tunnel: w539 -> [w563]
                  tunnel: w538 -> [w561]
                  tunnel: [w560] -> w537
                  tunnel: [w559] -> w536
                  tunnel: w535 -> [w558]
                  tunnel: [w557] -> w534
                  tunnel: w533 -> [w554]
                  tunnel: [w553] -> w532
                  tunnel: w531 -> [w551]
                  tunnel: 0 -> [w550]
                  tunnel: w529 -> [w548]
                  tunnel: [w544] -> w519 mode=indexing
                  tunnel: [w543] -> w527 mode=indexing
                  tunnel: [w542] -> w520 mode=indexing
                  i -> [w546]
                  stop <- w552 continue-if-true
                  n246 = Wait Until Next ms Multiple(millisecond multiple=w548) -> ()  [unwired: 1 out]
                  n247 = Bundle(w546, "step press (V)"=w551, w550) -> (w549:cluster{i32, "step press (V)":dbl, i32})  [unwired: 1 out]
                  n248 = flat-sequence {
                    tunnel: [w575] -> w564
                    tunnel: w563 -> [w575]
                    tunnel: [w574] -> w562
                    tunnel: w561 -> [w574]
                    tunnel: w558 -> [w573]
                    tunnel: [w572] -> w556
                    tunnel: [w571] -> w555
                    tunnel: w554 -> [w571]
                    tunnel: w549 -> [w570]
                    tunnel: [w569] -> w547
                    tunnel: w546 -> [w569]
                    tunnel: [w567] -> w545
                    tunnel: [w566] -> w541
                    tunnel: w565 -> [w597]
                    tunnel: w564 -> [w596]
                    tunnel: w562 -> [w595]
                    tunnel: [w593] -> w560
                    tunnel: [w592] -> w559
                    tunnel: [w581] -> w557
                    tunnel: w556 -> [w581]
                    tunnel: w555 -> [w590]
                    tunnel: [w589] -> w553
                    tunnel: [w585] -> w552
                    tunnel: w547 -> [_]
                    tunnel: w545 -> [w584]
                    tunnel: [w580] -> w544
                    tunnel: [w582] -> w543
                    tunnel: [w576] -> w542
                    tunnel: w541 -> [w576]
                    frame #0 {
                      n249 = local read "V max (V)"() -> (w568:dbl)
                      n250 = call "piezo-cluster.vi"("cluster carte entree"=w573, "cluster carte data"=w570) -> ("cluster carte sortie"=w572:T9, "voltage (V)"=w566:dbl)
                      "voltage stop (V)" <- w566
                      n251 = local write "voltage stop (V)"(w566) -> ()
                      n252 = Less?(x=w566, y=w568) -> (x < y?=w567:bool)
                    }
                    frame #1 {
                      n253 = local read "F contact (pN)"() -> (w587:dbl)
                      n254 = Tick Count (ms)() -> (millisecond timer value=w579:u32)
                      n255 = local read "t0"() -> (w578:u32)
                      n256 = call <vilib>:"IMAQdx Get Image.vi"("Buffer Number Mode (Next)"=IMAQdx_Buffer_Number_Mode."Next", "error in"=w595, "Image In"=w590, "Session In"=w596) -> ("error out"=w594:errorcluster, "Image Out"=w589:T3, "Session Out"=w591:T2)  [unwired: 1 in, 4 out]
                      n257 = Subtract(x=w579, y=w578) -> (x-y=w580:u32)
                      n258 = property class="IMAQdx"(reference=w591, error in=w594) -> (reference out=w593:T2, error out=w592:errorcluster, "LastBufferNumber"=w577:u32)
                      "derniere image" <- w577
                      n259 = call "fit-cluster.vi"("Image In"=w589, "donnees fit"=w597) -> ("F - baseline  (pN)"=w582:dbl)
                      n260 = local write "derniere image"(w577) -> ()
                      n261 = Absolute Value(x=w582) -> (abs(x)=w586:dbl)
                      n262 = Less?(x=w586, y=w587) -> (x < y?=w583:bool)
                      n263 = And(x=w583, y=w584) -> (x .and. y?=w585:bool)
                    }
                  }
                }
                n264 = local read "chemin complet position"() -> (w518:path)
                n265 = local read "chemin complet force"() -> (w525:path)
                n266 = Build Array(w519, w520) -> (w521:dbl[][])
                n267 = Build Array(w519, w527) -> (w526:dbl[][])
                n268 = call-poly <vilib>:"Write To Spreadsheet File.vi"("transpose? (no:F)"=TRUE, "append to file? (new file:F)"=TRUE, "2D data"=w521, "file path (dialog if empty)"=w518) -> ()  [unwired: 2 in, 3 out]
                n269 = call-poly <vilib>:"Write To Spreadsheet File.vi"("transpose? (no:F)"=TRUE, "append to file? (new file:F)"=TRUE, "2D data"=w526, "file path (dialog if empty)"=w525) -> ()  [unwired: 2 in, 3 out]
              }
              frame #5 {
                w611 = 2
                n270 = local read "t contact (s)"() -> (w607:dbl)
                n271 = Multiply(x=w607, y=1000) -> (x*y=w612:dbl)
                n272 = Divide(x=w612, y=w611) -> (x/y=w608:dbl)
                n273 = To Long Integer(number=w608) -> (32bit integer=w606:i32)
                n274 = Not Equal?(x=w608, y=0.0) -> (x != y?=w610:bool)
                n275 = case "si t=0 ou non" shown="True" w610 {
                  tunnel: w606 -> [_ w632]
                  tunnel: w611 -> [_ w629]
                  tunnel: w605 -> [w617 w640]
                  tunnel: w602 -> [_ w639]
                  tunnel: [w617 w638] -> w604
                  tunnel: [w616 w637] -> w603
                  tunnel: w602 -> [w616 _]
                  tunnel: w601 -> [w615 w636]
                  tunnel: [w615 w635] -> w600
                  tunnel: w599 -> [w614 w634]
                  tunnel: [w614 w633] -> w598
                  frame False {
                  }
                  frame True {
                    n276 = local read "voltage stop (V)"() -> (w630:dbl)
                    n277 = local read "cluster fit"() -> (w641:T1)
                    n278 = local read "chemin complet position"() -> (w618:path)
                    n279 = local read "chemin complet force"() -> (w625:path)
                    n280 = while {
                      tunnel: w641 -> [w667]
                      tunnel: w640 -> [w665]
                      tunnel: w639 -> [w663]
                      tunnel: [w662] -> w638
                      tunnel: [w661] -> w637
                      tunnel: w636 -> [w660]
                      tunnel: [w659] -> w635
                      tunnel: w634 -> [w656]
                      tunnel: [w655] -> w633
                      tunnel: w632 -> [w652]
                      tunnel: 0 -> [w651]
                      tunnel: w630 -> [w650]
                      tunnel: w629 -> [w648]
                      tunnel: [w645] -> w626 mode=indexing
                      tunnel: [w644] -> w619 mode=indexing
                      tunnel: [w643] -> w620 mode=indexing
                      i -> [w646]
                      stop <- w654 continue-if-true
                      n281 = Wait Until Next ms Multiple(millisecond multiple=w648) -> ()  [unwired: 1 out]
                      n282 = Bundle(w646, w651, "voltage stop (V)"=w650) -> (w649:cluster{i32, i32, "voltage stop (V)":dbl})  [unwired: 1 out]
                      n283 = flat-sequence {
                        tunnel: [w676] -> w666
                        tunnel: w665 -> [w676]
                        tunnel: [w675] -> w664
                        tunnel: w663 -> [w675]
                        tunnel: w660 -> [w674]
                        tunnel: [w673] -> w658
                        tunnel: [w672] -> w657
                        tunnel: w656 -> [w672]
                        tunnel: [w671] -> w653
                        tunnel: w652 -> [w671]
                        tunnel: w649 -> [w670]
                        tunnel: [w669] -> w647
                        tunnel: w646 -> [w669]
                        tunnel: [w668] -> w642
                        tunnel: w667 -> [w696]
                        tunnel: w666 -> [w695]
                        tunnel: w664 -> [w694]
                        tunnel: [w692] -> w662
                        tunnel: [w690] -> w661
                        tunnel: [w689] -> w659
                        tunnel: w658 -> [w689]
                        tunnel: w657 -> [w688]
                        tunnel: [w687] -> w655
                        tunnel: [w685] -> w654
                        tunnel: w646 -> [w683]
                        tunnel: w653 -> [w684]
                        tunnel: w647 -> [_]
                        tunnel: [w682] -> w645
                        tunnel: [w679] -> w644
                        tunnel: [w677] -> w643
                        tunnel: w642 -> [w677]
                        frame #0 {
                          n284 = call "piezo-cluster.vi"("cluster carte entree"=w674, "cluster carte data"=w670) -> ("cluster carte sortie"=w673:T9, "voltage (V)"=w668:dbl)
                        }
                        frame #1 {
                          n285 = Less?(x=w683, y=w684) -> (x < y?=w685:bool)
                          n286 = Tick Count (ms)() -> (millisecond timer value=w680:u32)
                          n287 = local read "t0"() -> (w681:u32)
                          n288 = call <vilib>:"IMAQdx Get Image.vi"("Buffer Number Mode (Next)"=IMAQdx_Buffer_Number_Mode."Next", "error in"=w694, "Image In"=w688, "Session In"=w695) -> ("error out"=w691:errorcluster, "Image Out"=w687:T3, "Session Out"=w693:T2)  [unwired: 1 in, 4 out]
                          n289 = Subtract(x=w680, y=w681) -> (x-y=w679:u32)
                          n290 = property class="IMAQdx"(reference=w693, error in=w691) -> (reference out=w692:T2, error out=w690:errorcluster, "LastBufferNumber"=w678:u32)
                          n291 = call "fit-cluster.vi"("Image In"=w687, "donnees fit"=w696) -> ("F - baseline  (pN)"=w682:dbl)
                          n292 = local write "derniere image"(w678) -> ()
                        }
                      }
                    }
                    n293 = Build Array(w619, w620) -> (w621:dbl[][])
                    n294 = Build Array(w619, w626) -> (w627:dbl[][])
                    n295 = call-poly <vilib>:"Write To Spreadsheet File.vi"("transpose? (no:F)"=TRUE, "append to file? (new file:F)"=TRUE, "2D data"=w621, "file path (dialog if empty)"=w618) -> ()  [unwired: 2 in, 3 out]
                    n296 = call-poly <vilib>:"Write To Spreadsheet File.vi"("transpose? (no:F)"=TRUE, "append to file? (new file:F)"=TRUE, "2D data"=w627, "file path (dialog if empty)"=w625) -> ()  [unwired: 2 in, 3 out]
                  }
                }
              }
              frame #6 {
              }
              frame #7 {
                n297 = local read "step pull  (ms)"() -> (w716:dbl)
                n298 = local read "cluster fit"() -> (w708:T1)
                n299 = local read "SD x"() -> (w701:dbl)
                n300 = while {
                  tunnel: w716 -> [w757]
                  tunnel: w718 -> [w741]
                  tunnel: [w758] -> w717
                  tunnel: [w756] -> w712 mode=indexing
                  tunnel: w710 -> [w755]
                  tunnel: w709 -> [w754]
                  tunnel: w708 -> [w753]
                  tunnel: [w752] -> w706 mode=indexing
                  tunnel: [w751] -> w707 mode=indexing
                  tunnel: w704 -> [w750]
                  tunnel: [w749] -> w703
                  tunnel: [w748] -> w702
                  tunnel: w701 -> [w722]
                  i -> [w725]
                  stop <- w747 continue-if-true
                  n301 = Wait Until Next ms Multiple(millisecond multiple=w757) -> ()  [unwired: 1 out]
                  n302 = flat-sequence {
                    tunnel: [w773] -> w739
                    tunnel: [w767] -> w737
                    tunnel: [w766] -> w735
                    tunnel: [w765] -> w733
                    tunnel: [w764] -> w730
                    tunnel: [w763] -> w728
                    tunnel: w750 -> [w768]
                    tunnel: w755 -> [w776]
                    tunnel: w754 -> [w775]
                    tunnel: w753 -> [w774]
                    tunnel: w741 -> [w764]
                    tunnel: w725 -> [w761]
                    tunnel: [w761] -> w724
                    tunnel: w722 -> [w759]
                    tunnel: w739 -> [w791]
                    tunnel: [w791] -> w738
                    tunnel: w737 -> [w790]
                    tunnel: [w790] -> w736
                    tunnel: w735 -> [w789]
                    tunnel: [w789] -> w734
                    tunnel: w733 -> [w786]
                    tunnel: [w785] -> w732
                    tunnel: [w783] -> w731
                    tunnel: w730 -> [w788]
                    tunnel: [w788] -> w729
                    tunnel: w728 -> [w787]
                    tunnel: [w787] -> w727
                    tunnel: w724 -> [w784]
                    tunnel: [w784] -> w723
                    tunnel: [w803] -> w746
                    tunnel: [w796] -> w745
                    tunnel: w738 -> [w806]
                    tunnel: [w806] -> w744
                    tunnel: w736 -> [w805]
                    tunnel: [w805] -> w743
                    tunnel: w734 -> [w804]
                    tunnel: [w804] -> w742
                    tunnel: w732 -> [w802]
                    tunnel: w731 -> [w801]
                    tunnel: w729 -> [w800]
                    tunnel: w727 -> [w799]
                    tunnel: [w799] -> w740
                    tunnel: [w796] -> w726
                    tunnel: w723 -> [w797]
                    tunnel: [w811] -> w749
                    tunnel: [w812] -> w748
                    tunnel: [w808] -> w751
                    tunnel: [w813] -> w752
                    tunnel: [w814] -> w756
                    tunnel: [w809] -> w747
                    tunnel: [w815] -> w758
                    tunnel: w746 -> [w815]
                    tunnel: w745 -> [w814]
                    tunnel: w744 -> [w813]
                    tunnel: w743 -> [w812]
                    tunnel: w742 -> [w811]
                    tunnel: w740 -> [w808]
                    tunnel: w726 -> [w807]
                    frame #0 {
                      n303 = local read "SD noise (pN)"() -> (w771:dbl)
                      n304 = Tick Count (ms)() -> (millisecond timer value=w782:u32)
                      n305 = local read "Clamp at (pN)"() -> (w762:dbl)
                      n306 = local read "t0"() -> (w781:u32)
                      n307 = Multiply(x=w771, y=w759) -> (x*y=w760:dbl)
                      n308 = call <vilib>:"IMAQdx Get Image.vi"("Buffer Number Mode (Next)"=IMAQdx_Buffer_Number_Mode."Next", "error in"=w768, "Image In"=w775, "Session In"=w776) -> ("error out"=w779:errorcluster, "Image Out"=w777:T3, "Session Out"=w778:T2)  [unwired: 1 in, 4 out]
                      n309 = Subtract(x=w782, y=w781) -> (x-y=w773:u32)
                      n310 = property class="IMAQdx"(reference=w778, error in=w779) -> (reference out=w767:T2, error out=w766:errorcluster, "LastBufferNumber"=w769:u32)
                      n311 = Add(x=w760, y=w762) -> (x+y=w772:dbl)
                      n312 = Subtract(x=w762, y=w760) -> (x-y=w770:dbl)
                      n313 = call "fit-cluster.vi"("Image In"=w777, "donnees fit"=w774) -> ("F - baseline  (pN)"=w763:dbl)
                      n314 = local write "derniere image"(w769) -> ()
                      n315 = In Range and Coerce(upper limit=w772, x=w763, lower limit=w770) -> (In Range?=w765:bool)  [unwired: 1 out]
                      n316 = local write "clamp test"(w765) -> ()
                    }
                    frame #1 {
                      n317 = local read "voltage stop (V)"() -> (w783:dbl)
                      n318 = case shown="False" w786 {
                        tunnel: [w792 w794] -> w785
                        frame False {
                          n319 = local read "step pull (V)"() -> (w793:dbl)
                          n320 = Negate(x=w793) -> (-x=w792:dbl)
                        }
                        frame True {
                          n321 = To Double Precision Float(number=0) -> (double precision float=w794:dbl)
                        }
                      }
                    }
                    frame #2 {
                      n322 = Bundle(w797, w802, "voltage stop (V)"=w801) -> (w798:cluster{i32, dbl, "voltage stop (V)":dbl})  [unwired: 1 out]
                      n323 = call "piezo-cluster-clamp.vi"("cluster carte entree"=w800, "cluster carte data"=w798) -> ("cluster carte sortie"=w803:T9, "voltage (V)"=w796:dbl)
                      n324 = local write "voltage stop (V)"(w796) -> ()
                    }
                    frame #3 {
                      n325 = Greater?(x=w807, y=0) -> (0:w809:bool)
                    }
                  }
                  n326 = local write "test fin"(w747) -> ()
                  "test fin" <- w747
                }
                n327 = local read "chemin complet position"() -> (w713:path)
                n328 = local read "chemin complet force"() -> (w720:path)
                n329 = Build Array(w706, w712) -> (w711:dbl[][])
                n330 = Build Array(w706, w707) -> (w705:dbl[][])
                n331 = call-poly <vilib>:"Write To Spreadsheet File.vi"("transpose? (no:F)"=TRUE, "append to file? (new file:F)"=TRUE, "2D data"=w711, "file path (dialog if empty)"=w713) -> ()  [unwired: 2 in, 3 out]
                n332 = call-poly <vilib>:"Write To Spreadsheet File.vi"("transpose? (no:F)"=TRUE, "append to file? (new file:F)"=TRUE, "2D data"=w705, "file path (dialog if empty)"=w720) -> ()  [unwired: 2 in, 3 out]
              }
              frame #8 {
                n333 = local read "chemin complet force"() -> (w824:path)
                n334 = call-poly <vilib>:"Read From Spreadsheet File.vi"("transpose (no:F)"=TRUE, "number of rows (all:-1)"=-1, "file path (dialog if empty)"=w824) -> ("all rows"=w819:dbl[][])  [unwired: 1 in, 7 out]
                n335 = call "Convertir en données dynamiques"("2D Array"=w819) -> ("Dynamic Data Type"=w823:dynamicdata)  [unwired: 3 out]
                n336 = Split Signals(w823) -> (w822:dynamicdata, w821:dynamicdata)  [unwired: 2 out]
                n337 = call "Construire un graphe XY"("Reset"=TRUE, "Y Input"=w821, "X Input"=w822) -> ("XY Graph"=→"Data":cluster{"Y":dbl[], "Y":dbl[]}[])  [unwired: 2 in, 6 out]
              }
            }
          }
        }
        frame #2 {
          n338 = Unbundle(w832) -> ("task out"=w831:refnum<k21>, "error out"=w830:errorcluster)
          n339 = call <vilib>:"IMAQdx Close Camera.vi"("error in"=w829, "Session In"=w828) -> ("error out"=w833:errorcluster)  [unwired: 9 out]
          n340 = call <vilib>:"DAQmx Stop Task.vi"("task/channels in"=w831, "error in"=w830) -> ()  [unwired: 14 out]
          n341 = call <vilib>:"Simple Error Handler.vi"("error in (no error)"=w833) -> ()  [unwired: 1 in, 8 out]
        }
      }
    }
  }
